vi "Unflatten Payload.vi"(8 "error in":errorcluster, 11 "QMHMessagePayload in":refnum<class "QMHMessagePayload.lvclass">) -> (0 "error out":errorcluster, 2 "Payload":variant, 3 "QMHMessagePayload out":refnum<class "QMHMessagePayload.lvclass">)   [LabVIEW 2016, in "QMHMessagePayload.lvclass"]
uses:
  QMHMessagePayload.lvclass
  QMHMessagePayload.lvclass/QMHMessagePayload.ctl
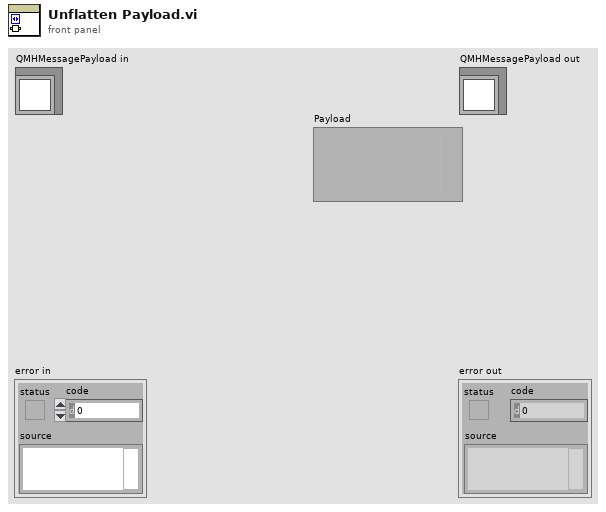
[diagram p1: front panel]
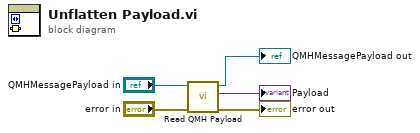
[diagram p0: block diagram]
diagram:
  n1 = call "Read QMH Payload.vi"("error in (no error)"="error in", "QMHMessagePayload in"="QMHMessagePayload in") -> ("error out"=→"error out":errorcluster, "QMH Payload"=→"Payload":variant, "QMHMessagePayload out"=→"QMHMessagePayload out":refnum<class "QMHMessagePayload.lvclass">)  [unwired: 7 in]
